vi "get shot numbers from tcp array.vi"(11 "element":string[][](array[string])) -> (3 "Shotnumbers":i32[](array[numeric]))   [LabVIEW 2020]
panel:
  out "Shotnumbers strings":string[](array[string])
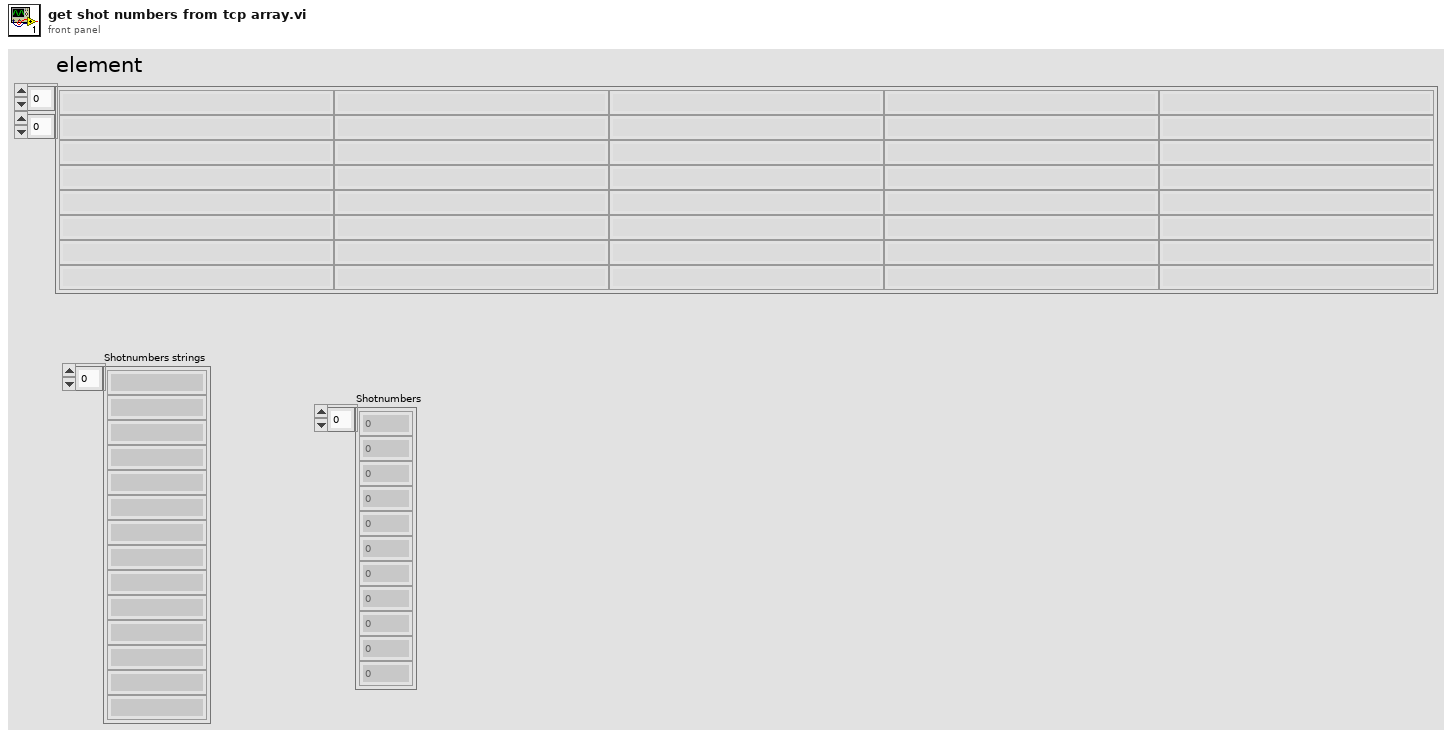
[diagram p1: front panel]
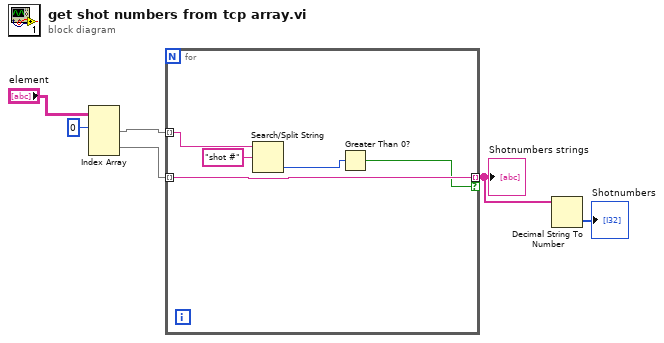
[diagram p0: block diagram]
diagram:
  n1 = Index Array(array="element", index (row) #1=0 ("index (row)")) -> (element #1=w4:string[], element #2=w3:string[])  [unwired: 3 in]
  n2 = for {
    tunnel: w4 -> [w11] mode=indexing
    tunnel: w3 -> [w9] mode=indexing
    tunnel: [w9] -> w2 mode=indexing if=w7
    n3 = Search/Split String(string=w11, search string/char (-)="shot #") -> (offset of match=w8:i32)  [unwired: 1 in, 2 out]
    n4 = Greater Than 0?(x=w8) -> (x > 0?=w7:bool)
  }
  "Shotnumbers strings" <- w2
  n5 = Decimal String To Number(string=w2) -> (number=→"Shotnumbers":i32[])  [unwired: 2 in, 1 out]
